vi "KCube_IsActiveAndActivate.vi"(11 "KCubePiezoDevice Z Reference":refnum<k24>) -> (1 "IsSetOutputVoltageActive":bool, 2 "reference out":refnum<k24>, 3 "GetOutputVoltage":dbl)   [LabVIEW 2019]
uses:
  C:/Users/manip/Documents/Controle_Manip_2020/Thorlabs.MotionControl.KCube.PiezoCLI.dll
  Thorlabs.MotionControl.KCube.PiezoCLI.dll
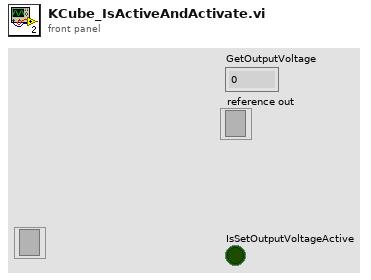
[diagram p1: front panel]
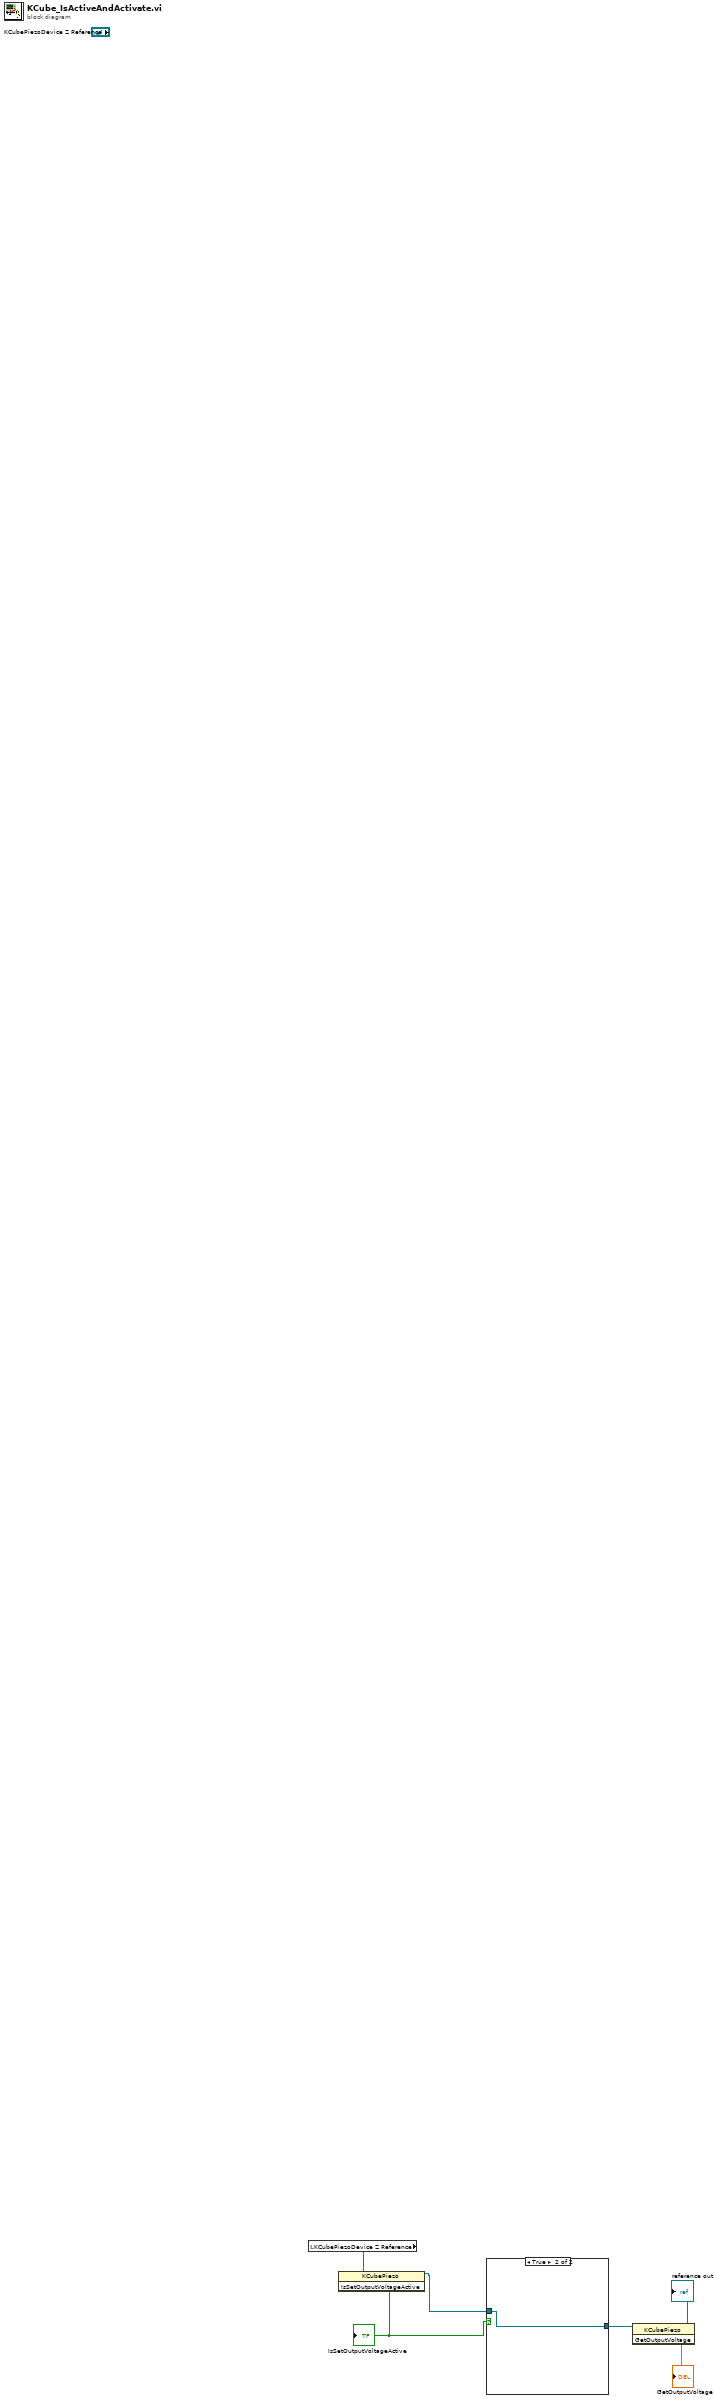
[diagram p0: block diagram]
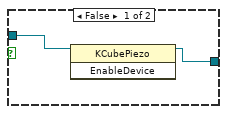
[diagram p2: hidden frame]
diagram:
  n1 = local read "KCubePiezoDevice Z Reference"() -> (w6:refnum<k24>)
  n2 = invoke class="KCubePiezo" method="IsSetOutputVoltageActive"(reference=w6) -> (reference out=w4:refnum<k24>, "IsSetOutputVoltageActive"=w5:bool)  [unwired: 2 in, 1 out]
  "IsSetOutputVoltageActive" <- w5
  n3 = case shown="True" w5 {
    tunnel: w4 -> [w8 w9]
    tunnel: [w7 w9] -> w3
    frame False {
      n4 = invoke class="KCubePiezo" method="EnableDevice"(reference=w8) -> (reference out=w7:refnum<k24>)  [unwired: 2 in, 2 out]
    }
    frame True {
    }
  }
  n5 = invoke class="KCubePiezo" method="GetOutputVoltage"(reference=w3) -> (reference out=→"reference out":refnum<k24>, "GetOutputVoltage"=→"GetOutputVoltage":dbl)  [unwired: 2 in, 1 out]
